vi "Exercise1.5-Array and Cluster.vi"() -> ()   [LabVIEW 2013]
panel:
  out "Cluster":T1
  out "String Array":string[](array[string])
  out "Boolean Array":bool[](array[boolean])
  in  "Numeric Array":dbl[](array[numeric])
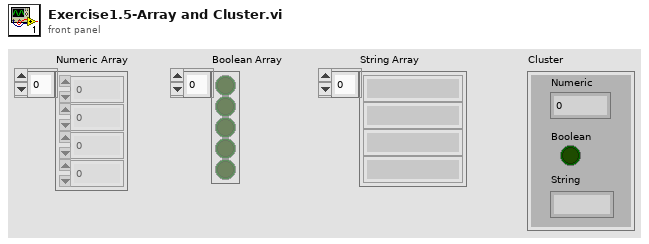
[diagram p1: front panel]
types:
  T1 = cluster{"Numeric":dbl, "Boolean":bool, "String":string}
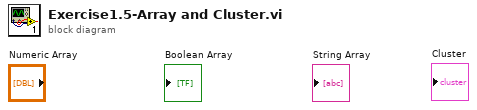
[diagram p0: block diagram]
diagram:
